vi "sub_SDR_demod_bitsToString.vi"(10 "Input bits":bool[](array[boolean])) -> (2 "Output string":string)   [LabVIEW 2012]
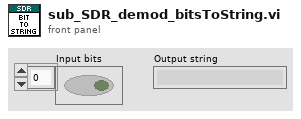
[diagram p1: front panel]
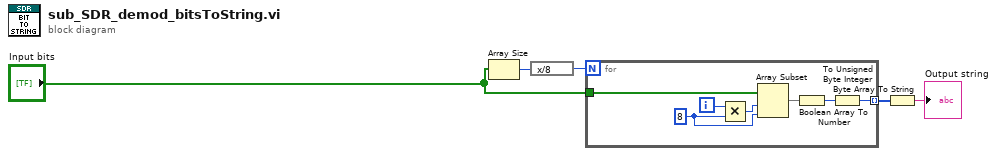
[diagram p0: block diagram]
diagram:
  n1 = Array Size(array="Input bits") -> (size(s)=w3:i32)
  n2 = expression code="x/8"(w3) -> (w2:i32)
  n3 = for {
    N: w2 -> [_]
    tunnel: "Input bits" -> [w12]
    tunnel: [w7] -> w4 mode=indexing
    i -> [w10]
    w9 = 8 ("length")
    n4 = Multiply(x=w10, y=w9) -> (x*y=w11:i32)
    n5 = Array Subset(array=w12, index=w11, length=w9) -> (w6:bool[])
    n6 = Boolean Array To Number(Boolean array=w6) -> (number=w8:u32)
    n7 = To Unsigned Byte Integer(number=w8) -> (unsigned 8bit integer=w7:u8)
  }
  n8 = Byte Array To String(unsigned byte array=w4) -> (string=→"Output string":string)
